vi "Chat_main.vi"() -> ()   [LabVIEW 2011]
uses:
  Controls/Stage.ctl
panel:
  in  "Port":u16=13078
  in  "Host IP":string="127.0.0.1"
  out "OnlineList":string[](array[string])
  in  "Create":bool
  in  "OffLine":bool
  in  "Link":bool
  out "linked":bool
  in  "Nickname":string
  in  "Send":bool
  in  "MsgBox":string
  out "C_Room":string
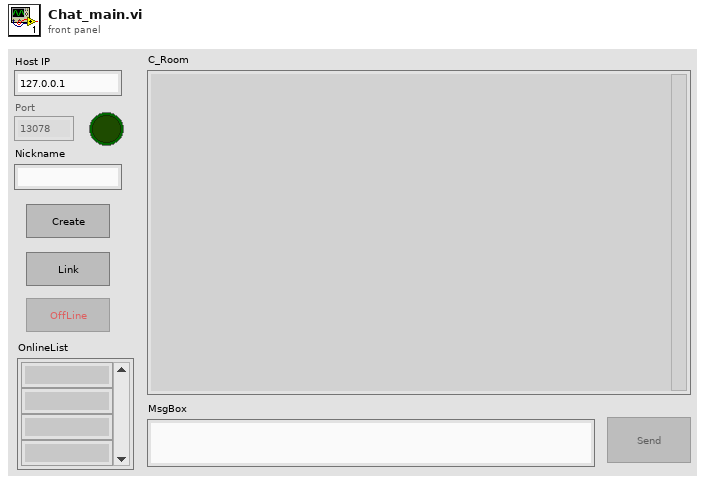
[diagram p1: front panel]
types:
  T1 = typedef "Stage.ctl" = enum16{"Initial", "Idle", "Link", "TX", "RX", "stop"}
  T2 = enum8{"Enabled", "Disabled", "Disabled and Grayed Out"}
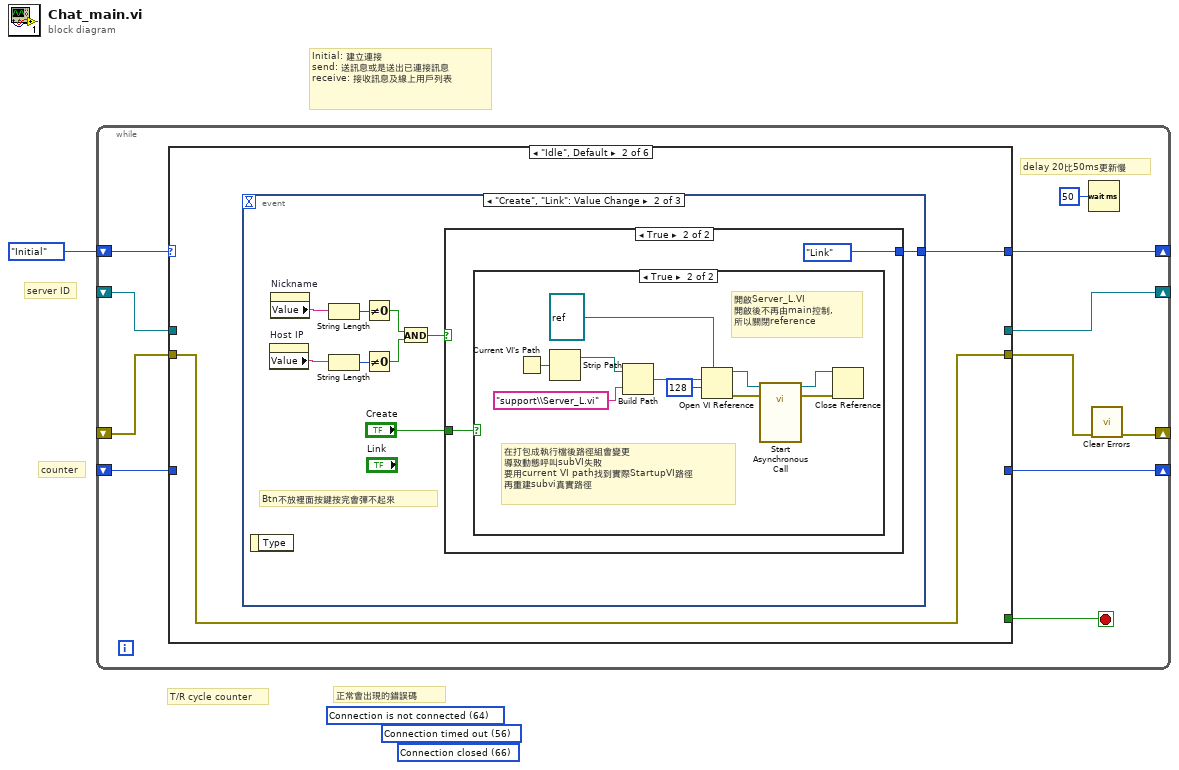
[diagram p0: block diagram]
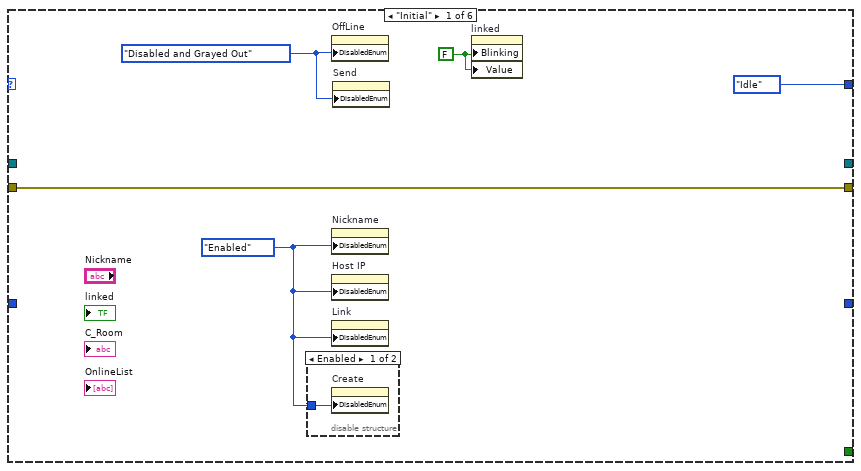
[diagram p2: hidden frame]
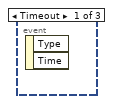
[diagram p4: hidden frame]
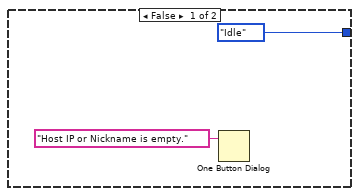
[diagram p5: hidden frame]
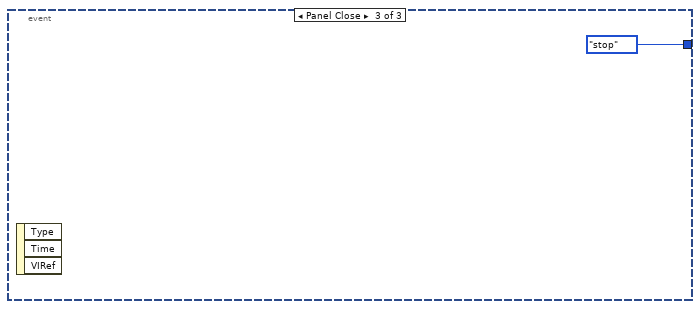
[diagram p7: hidden frame]
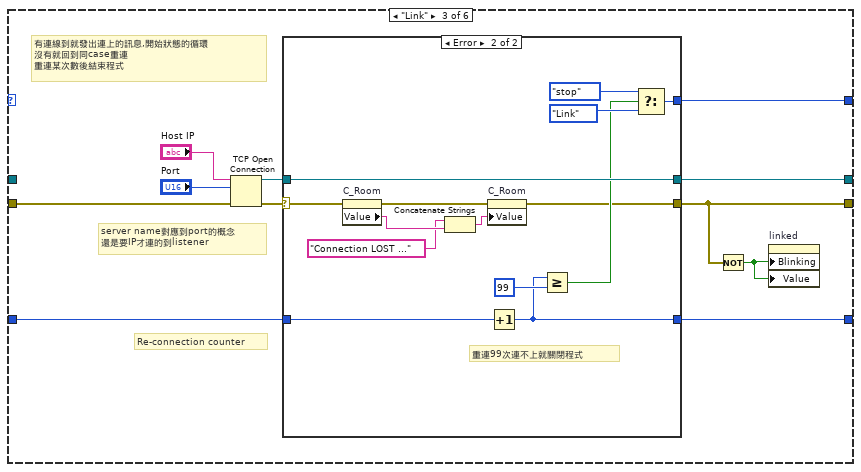
[diagram p8: hidden frame]
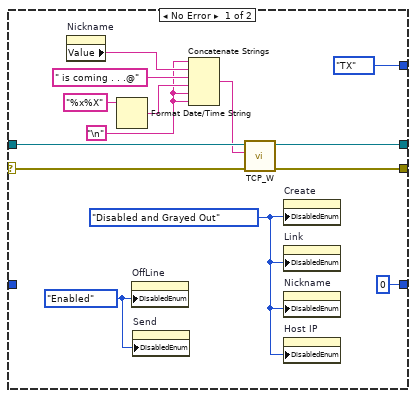
[diagram p9: hidden frame]
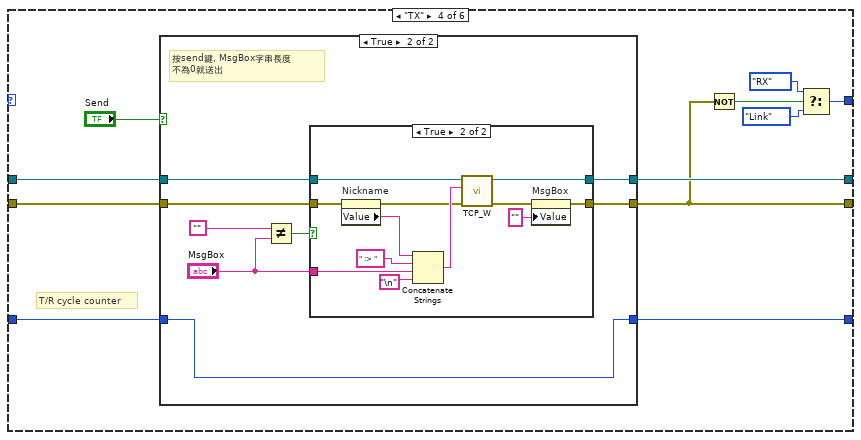
[diagram p10: hidden frame]
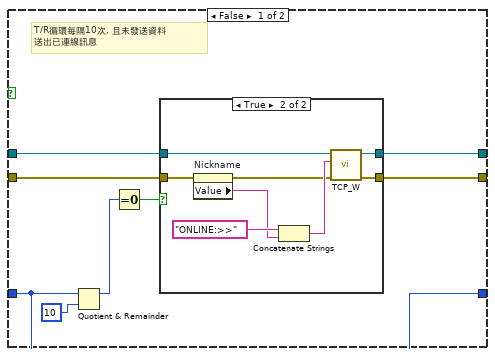
[diagram p11: hidden frame]
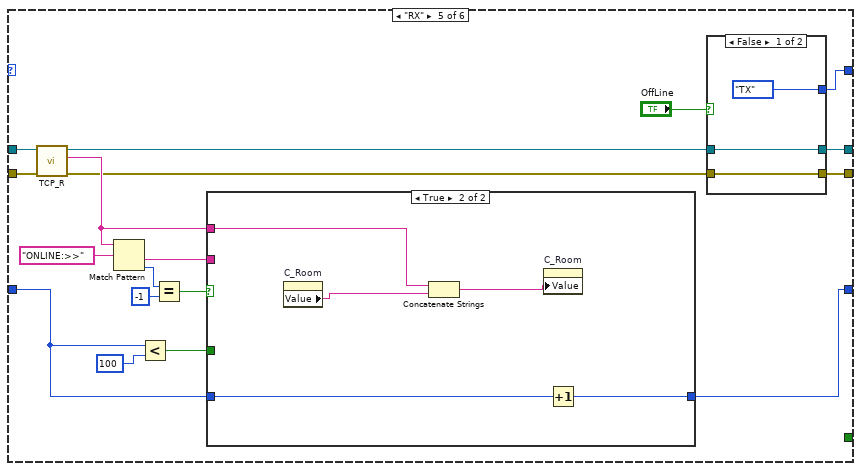
[diagram p14: hidden frame]
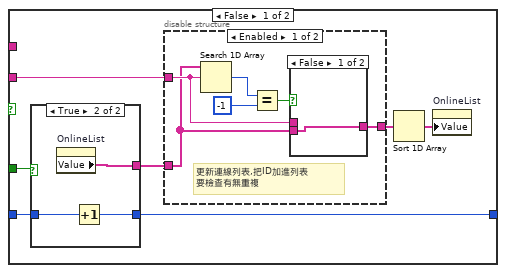
[diagram p15: hidden frame]
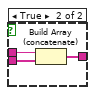
[diagram p16: hidden frame]
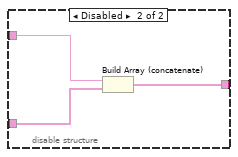
[diagram p17: hidden frame]
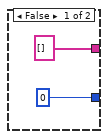
[diagram p18: hidden frame]
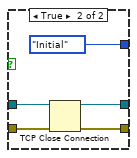
[diagram p19: hidden frame]
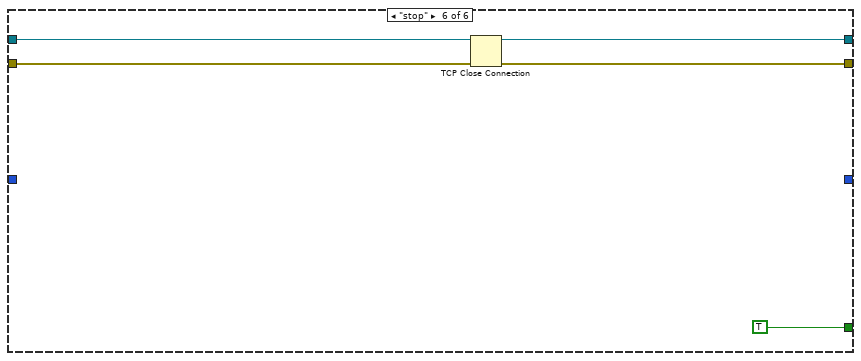
[diagram p20: hidden frame]
diagram:
  (unwired) 56 items=["No Error", "Argument Error", "Memory Full", "Out of Zone", "End of File", "File Already Open", "Generic File IO Error", "File Not Found", "File Permission Error", "Disk Full", "Duplicate Path", "Too Many Files Open", "Not Enabled", "Resource File Not Found", "Cannot Add Resource", "Resource Not Found", "Image Not Found", "Image Memory Error", "Pen Does Not Exist", "Config Bad Type", "Config Token Not Found", "Config Parse Error", "Config Memory Error", "Bad External Code Format", "Bad External Code Offset", "External Code Not Present", "Null Window", "Destroy Window Mixup", "Null Menu", "Print Aborted", "Bad Print Record", "Print Driver Error", "Windows Error During Print", "Memory Error During Print", "Print Dialog Error", "Generic Print Error", "Invalid Device Refnum", "Device Not Found", "Device Parameter Error", "Device Unit Error", "Can't Open Device", "Device Call Aborted", "Generic Error", "Cancelled By User", "Object ID Too Low", "Object ID Too High", "Object Not In Heap", "Unknown Heap", "Bad DefProc ID", "DefProc Not In Table", "Message Out Of Range", "Null Method", "Unknown Message", "Manager Call Not Supported", "Bad address", "Connection In progress", "Connection timed out", "Connection is already in progress", "Network attribute not supported", "Network error", "Address in use", "System out of memory", "Connection aborted", "Connection refused", "Connection is not connected", "Connection is already connected", "Connection closed", "Initialize error (interapplication manager)", "Bad occurrence", "Wait on unbound occurrence handler", "Occurrence queue overflow", "Bad path", "Semaphore not signaled", "Unrecognized type (interapplication manager)"] ("2nd Error to Convert")
  (unwired) 66 items=["No Error", "Argument Error", "Memory Full", "Out of Zone", "End of File", "File Already Open", "Generic File IO Error", "File Not Found", "File Permission Error", "Disk Full", "Duplicate Path", "Too Many Files Open", "Not Enabled", "Resource File Not Found", "Cannot Add Resource", "Resource Not Found", "Image Not Found", "Image Memory Error", "Pen Does Not Exist", "Config Bad Type", "Config Token Not Found", "Config Parse Error", "Config Memory Error", "Bad External Code Format", "Bad External Code Offset", "External Code Not Present", "Null Window", "Destroy Window Mixup", "Null Menu", "Print Aborted", "Bad Print Record", "Print Driver Error", "Windows Error During Print", "Memory Error During Print", "Print Dialog Error", "Generic Print Error", "Invalid Device Refnum", "Device Not Found", "Device Parameter Error", "Device Unit Error", "Can't Open Device", "Device Call Aborted", "Generic Error", "Cancelled By User", "Object ID Too Low", "Object ID Too High", "Object Not In Heap", "Unknown Heap", "Bad DefProc ID", "DefProc Not In Table", "Message Out Of Range", "Null Method", "Unknown Message", "Manager Call Not Supported", "Bad address", "Connection In progress", "Connection timed out", "Connection is already in progress", "Network attribute not supported", "Network error", "Address in use", "System out of memory", "Connection aborted", "Connection refused", "Connection is not connected", "Connection is already connected", "Connection closed", "Initialize error (interapplication manager)", "Bad occurrence", "Wait on unbound occurrence handler", "Occurrence queue overflow", "Bad path", "Semaphore not signaled", "Unrecognized type (interapplication manager)"] ("3rd Error to Convert")
  (unwired) 64 items=["No Error", "Argument Error", "Memory Full", "Out of Zone", "End of File", "File Already Open", "Generic File IO Error", "File Not Found", "File Permission Error", "Disk Full", "Duplicate Path", "Too Many Files Open", "Not Enabled", "Resource File Not Found", "Cannot Add Resource", "Resource Not Found", "Image Not Found", "Image Memory Error", "Pen Does Not Exist", "Config Bad Type", "Config Token Not Found", "Config Parse Error", "Config Memory Error", "Bad External Code Format", "Bad External Code Offset", "External Code Not Present", "Null Window", "Destroy Window Mixup", "Null Menu", "Print Aborted", "Bad Print Record", "Print Driver Error", "Windows Error During Print", "Memory Error During Print", "Print Dialog Error", "Generic Print Error", "Invalid Device Refnum", "Device Not Found", "Device Parameter Error", "Device Unit Error", "Can't Open Device", "Device Call Aborted", "Generic Error", "Cancelled By User", "Object ID Too Low", "Object ID Too High", "Object Not In Heap", "Unknown Heap", "Bad DefProc ID", "DefProc Not In Table", "Message Out Of Range", "Null Method", "Unknown Message", "Manager Call Not Supported", "Bad address", "Connection In progress", "Connection timed out", "Connection is already in progress", "Network attribute not supported", "Network error", "Address in use", "System out of memory", "Connection aborted", "Connection refused", "Connection is not connected", "Connection is already connected", "Connection closed", "Initialize error (interapplication manager)", "Bad occurrence", "Wait on unbound occurrence handler", "Occurrence queue overflow", "Bad path", "Semaphore not signaled", "Unrecognized type (interapplication manager)"] ("1st Error to Convert")
  # "正常會出現的錯誤碼"
  # "T/R cycle counter"
  # "server ID"
  # "counter"
  # "Initial: 建立連接\nsend: 送訊息或是送出已連接訊息\nreceive: 接收訊息及線上用戶列表"
  n1 = while {
    shift-right: [w11] -> _
    shift-left: Stage."Initial" -> [w12]
    shift-right: [w9] -> _
    shift-left: _ -> [w8]
    shift-right: [w2] -> _
    shift-left: _ -> [w7]
    shift-right: [w4] -> _
    shift-left: _ -> [w5]
    stop <- w10 stop-if-true
    # "delay 20比50ms更新慢"
    n2 = case shown="\"Idle\", Default" w12 {
      tunnel: [Stage."Idle" w20 w52 w89 w147 _] -> w11
      tunnel: [_ _ _ _ _ TRUE ("stop")] -> w10
      tunnel: [_ _ w54 w93 w148 w191] -> w9
      tunnel: w8 -> [_ _ _ w94 w152 w194]
      tunnel: [w14 w19 w47 w84 w146 w193] -> w3
      tunnel: w7 -> [w14 w19 w48 w92 w151 w192]
      tunnel: w5 -> [_ _ w51 w86 w138 _]
      tunnel: [_ _ w50 w85 w140 _] -> w4
      frame "Initial" {
        w13 = T2."Enabled" ("Disabled")
        w15 = FALSE ("Link")
        w16 = T2."Disabled and Grayed Out" ("Disabled")
        n3 = disable-structure shown="Enabled" {
          disable-tunnel: w13 -> [w18 _]
          frame Enabled {
            n4 = property on="Create" class="Bool"("DisabledEnum"=w18) -> ()  [unwired: 2 in, 2 out]
          }
          frame Disabled {
          }
        }
        n5 = property on="OffLine" class="Bool"("DisabledEnum"=w16) -> ()  [unwired: 2 in, 2 out]
        n6 = property on="Nickname" class="Str"("DisabledEnum"=w13) -> ()  [unwired: 2 in, 2 out]
        n7 = property on="Host IP" class="Str"("DisabledEnum"=w13) -> ()  [unwired: 2 in, 2 out]
        n8 = property on="Link" class="Bool"("DisabledEnum"=w13) -> ()  [unwired: 2 in, 2 out]
        n9 = property on="Send" class="Bool"("DisabledEnum"=w16) -> ()  [unwired: 2 in, 2 out]
        n10 = property on="linked" class="Bool (strict)"("Blinking"=w15, "Value"=w15) -> ()  [unwired: 2 in, 2 out]
      }
      frame "Idle", Default {
        n11 = event shown="[1] \"Create\", \"Link\": Value Change" {
          selector: _ -> [_ _ _]
          dyn-events: _ -> [_ _ _]
          timeout: _ -> [_ _ _]
          tunnel: [_ w29 Stage."stop"] -> w20
          event Timeout {
            n12 = event-data() -> ()  [unwired: 1 in, 2 out]
          }
          event "Create", "Link": Value Change {
            # "Btn不放裡面按鍵按完會彈不起來"
            n13 = event-data() -> ()  [unwired: 1 in, 1 out]
            n14 = property on="Host IP" class="Str"() -> ("Value"=w22:string)  [unwired: 2 in, 2 out]
            n15 = property on="Nickname" class="Str"() -> ("Value"=w25:string)  [unwired: 2 in, 2 out]
            n16 = String Length(string=w25) -> (length=w28:i32)
            n17 = String Length(string=w22) -> (length=w26:i32)
            n18 = Not Equal To 0?(x=w28) -> (x != 0?=w24:bool)
            n19 = Not Equal To 0?(x=w26) -> (x != 0?=w23:bool)
            n20 = And(x=w24, y=w23) -> (x .and. y?=w27:bool)
            n21 = case shown="True" w27 {
              tunnel: [Stage."Idle" Stage."Link"] -> w29
              tunnel: "Create" -> [_ w32]
              frame False {
                n22 = One Button Dialog(message="Host IP or Nickname is empty.") -> ()  [unwired: 1 in, 1 out]
              }
              frame True {
                n23 = case shown="True" w32 {
                  frame False {
                  }
                  frame True {
                    # "在打包成執行檔後路徑組會變更\n導致動態呼叫subVI失敗\n要用current VI path找到實際StartupVI路徑\n再重建subvi真實路徑"
                    # "開啟Server_L.VI\n開啟後不再由main控制,\n所以關閉reference"
                    n24 = Current VI's Path() -> (path=w35:path)
                    n25 = Strip Path(path=w35) -> (stripped path=w34:path)  [unwired: 1 out]
                    n26 = Build Path(base path=w34, name or relative path="support\\Server_L.vi" ("vi path")) -> (appended path=w39:path)
                    n27 = Open VI Reference(type specifier VI Refnum (for type only)=refnum<vi> refnum, vi path=w39, options=128) -> (vi reference=w43:refnum<vi>, error out=w41:errorcluster)  [unwired: 3 in]
                    n28 = call-by-ref "Start Asynchronous Call"(reference=w43, error in=w41) -> (reference out=w36:refnum<vi>, error out=w37:errorcluster)  [unwired: 12 in]
                    n29 = Close Reference(reference=w36, error in (no error)=w37) -> ()  [unwired: 1 out]
                  }
                }
              }
            }
          }
          event Panel Close {
            n30 = event-data() -> ()  [unwired: 1 in, 3 out]
          }
        }
      }
      frame "Link" {
        # "Re-connection counter"
        # "server name對應到port的概念\n還是要IP才連的到listener"
        # "有連線到就發出連上的訊息,開始狀態的循環\n沒有就回到同case重連\n重連某次數後結束程式"
        n31 = TCP Open Connection(address="Host IP", remote port or service name="Port", error in (no error)=w48) -> (connection ID=w55:refnum<k5>, error out=w53:errorcluster)  [unwired: 2 in]
        n32 = case shown="Error" w53 {
          selector: w53 -> [w68 w73]
          tunnel: [w58 w71] -> w47
          tunnel: w55 -> [w69 w83]
          tunnel: [w59 w83] -> w54
          tunnel: [Stage."TX" w81] -> w52
          tunnel: w51 -> [_ w82]
          tunnel: [0 w77] -> w50
          frame No Error {
            w57 = T2."Disabled and Grayed Out" ("Disabled")
            w60 = T2."Enabled" ("Disabled")
            w56 = "\n"
            n33 = property on="Nickname" class="Str"() -> ("Value"=w61:string)  [unwired: 2 in, 2 out]
            n34 = Format Date/Time String(time format string (%c)="%x%X") -> (date/time string=w62:string)  [unwired: 2 in]
            n35 = property on="OffLine" class="Bool"("DisabledEnum"=w60) -> ()  [unwired: 2 in, 2 out]
            n36 = property on="Send" class="Bool"("DisabledEnum"=w60) -> ()  [unwired: 2 in, 2 out]
            n37 = Concatenate Strings(w56, w61, " is coming . . .@" ("data in"), w62, w56, w56) -> (w64:string)
            n38 = call "TCP_W.vi"("error in"=w68, "data in"=w64, "connection ID"=w69) -> ("error IO"=w58:errorcluster, "connection ID out"=w59:refnum<k5>)  [unwired: 7 in]
            n39 = property on="Create" class="Bool"("DisabledEnum"=w57) -> ()  [unwired: 2 in, 2 out]
            n40 = property on="Link" class="Bool"("DisabledEnum"=w57) -> ()  [unwired: 2 in, 2 out]
            n41 = property on="Nickname" class="Str"("DisabledEnum"=w57) -> ()  [unwired: 2 in, 2 out]
            n42 = property on="Host IP" class="Str"("DisabledEnum"=w57) -> ()  [unwired: 2 in, 2 out]
          }
          frame Error {
            # "重連99次連不上就關閉程式"
            n43 = property on="C_Room" class="Str"(error in=w73) -> (error out=w72:errorcluster, "Value"=w74:string)  [unwired: 1 in, 1 out]
            n44 = Concatenate Strings("Connection LOST ..." ("string"), w74) -> (w75:string)
            n45 = property on="C_Room" class="Str"(error in=w72, "Value"=w75) -> (error out=w71:errorcluster)  [unwired: 1 in, 1 out]
            n46 = Increment(x=w82) -> (x+1=w77:i32)
            n47 = Greater Or Equal?(x=w77, y=99) -> (x >= y?=w76:bool)
            n48 = Select(t=Stage."stop", s=w76, f=Stage."Link") -> (s? t:f=w81:T1)
          }
        }
        n49 = Not(x=w47) -> (.not. x?=w49:bool)
        n50 = property on="linked" class="Bool (strict)"("Blinking"=w49, "Value"=w49) -> ()  [unwired: 2 in, 2 out]
      }
      frame "TX" {
        # "T/R cycle counter"
        n51 = case shown="True" "Send" {
          tunnel: w94 -> [w102 w119]
          tunnel: [w101 w118] -> w93
          tunnel: w92 -> [w100 w120]
          tunnel: [w99 w117] -> w84
          tunnel: w86 -> [w95 w116]
          tunnel: [w95 w116] -> w85
          frame False {
            # "T/R循環每隔10次, 且未發送資料\n送出已連線訊息"
            n52 = Quotient & Remainder(x=w95, y=10) -> (x-y*floor(x/y)=w98:i32)  [unwired: 1 out]
            n53 = Equal To 0?(x=w98) -> (x = 0?=w96:bool)
            n54 = case shown="True" w96 {
              tunnel: w102 -> [w103 w112]
              tunnel: [w103 w111] -> w101
              tunnel: w100 -> [w104 w106]
              tunnel: [w104 w110] -> w99
              frame False {
              }
              frame True {
                n55 = property on="Nickname" class="Str"(error in=w106) -> (error out=w105:errorcluster, "Value"=w107:string)  [unwired: 1 in, 1 out]
                n56 = Concatenate Strings("ONLINE:>>" ("data in"), w107) -> (w108:string)
                n57 = call "TCP_W.vi"("error in"=w105, "data in"=w108, "connection ID"=w112) -> ("error IO"=w110:errorcluster, "connection ID out"=w111:refnum<k5>)  [unwired: 7 in]
              }
            }
          }
          frame True {
            # "按send鍵, MsgBox字串長度\n不為0就送出"
            n58 = Not Equal?(x="", y="MsgBox") -> (x != y?=w113:bool)
            n59 = case shown="True" w113 {
              tunnel: w119 -> [w121 w131]
              tunnel: w120 -> [w122 w124]
              tunnel: [w122 w128] -> w117
              tunnel: "MsgBox" -> [_ w126]
              tunnel: [w121 w125] -> w118
              frame False {
              }
              frame True {
                n60 = property on="Nickname" class="Str"(error in=w124) -> (error out=w123:errorcluster, "Value"=w127:string)  [unwired: 1 in, 1 out]
                n61 = Concatenate Strings(w127, " :> ", w126, "\n") -> (w132:string)
                n62 = call "TCP_W.vi"("error in"=w123, "data in"=w132, "connection ID"=w131) -> ("error IO"=w129:errorcluster, "connection ID out"=w125:refnum<k5>)  [unwired: 7 in]
                n63 = property on="MsgBox" class="Str"(error in=w129, "Value"="" ("MsgBox")) -> (error out=w128:errorcluster)  [unwired: 1 in, 1 out]
              }
            }
          }
        }
        n64 = Not(x=w84) -> (.not. x?=w88:bool)
        n65 = Select(t=Stage."RX", s=w88, f=Stage."Link") -> (s? t:f=w89:T1)
      }
      frame "RX" {
        n66 = call "TCP_R.vi"("error in"=w151, "connection ID"=w152) -> ("error out"=w135:errorcluster, "data out"=w136:string, "connection ID out"=w149:refnum<k5>)  [unwired: 7 in]
        n67 = Match Pattern(string=w136, regular expression="ONLINE:>>") -> (after substring=w141:string, offset past match=w142:i32)  [unwired: 1 in, 2 out]
        n68 = Less?(x=w138, y=100) -> (x < y?=w137:bool)
        n69 = Equal?(x=w142, y=-1 ("offset (0)")) -> (x = y?=w143:bool)
        n70 = case shown="True" w143 {
          tunnel: w136 -> [_ w180]
          tunnel: w141 -> [w159 _]
          tunnel: w138 -> [w155 w181]
          tunnel: [w158 w182] -> w140
          tunnel: w137 -> [w154 _]
          frame False {
            n71 = case shown="True" w154 {
              tunnel: [0 ("t") w177] -> w158
              tunnel: [string[] [] ("OnlineList") w175] -> w157
              tunnel: w155 -> [_ w176]
              frame False {
              }
              frame True {
                n72 = property on="OnlineList" class="Arr (strict)"() -> ("Value"=w175:string[])  [unwired: 2 in, 2 out]
                n73 = Increment(x=w176) -> (x+1=w177:i32)
              }
            }
            n74 = disable-structure shown="Enabled" {
              disable-tunnel: w159 -> [w162 w172]
              disable-tunnel: w157 -> [w161 w171]
              disable-tunnel: [w160 w170] -> w156
              frame Enabled {
                # "更新連線列表,把ID加進列表\n要檢查有無重複"
                n75 = Search 1D Array(1D array=w161, element=w162) -> (index of element=w163:i32)  [unwired: 1 in]
                n76 = Equal?(x=w163, y=-1) -> (x = y?=w164:bool)
                n77 = case shown="False" w164 {
                  tunnel: [w166 w169] -> w160
                  tunnel: w162 -> [_ w168]
                  tunnel: w161 -> [w166 w167]
                  frame False {
                  }
                  frame True {
                    n78 = Build Array (concatenate)(w168, w167) -> (w169:string[])
                  }
                }
              }
              frame Disabled {
                n79 = Build Array (concatenate)(w172, w171) -> (w170:string[])
              }
            }
            n80 = Sort 1D Array(array=w156) -> (sorted array=w153:string[])
            n81 = property on="OnlineList" class="Arr (strict)"("Value"=w153) -> ()  [unwired: 2 in, 2 out]
          }
          frame True {
            n82 = property on="C_Room" class="Str"() -> ("Value"=w178:string)  [unwired: 2 in, 2 out]
            n83 = Concatenate Strings(w180, w178) -> (w179:string)
            n84 = property on="C_Room" class="Str"("Value"=w179) -> ()  [unwired: 2 in, 2 out]
            n85 = Increment(x=w181) -> (x+1=w182:i32)
          }
        }
        n86 = case shown="False" "OffLine" {
          tunnel: [Stage."TX" Stage."Initial"] -> w147
          tunnel: w149 -> [w184 w189]
          tunnel: [w184 w188] -> w148
          tunnel: [w183 w187] -> w146
          tunnel: w135 -> [w183 w186]
          frame False {
          }
          frame True {
            n87 = TCP Close Connection(connection ID=w189, error in (no error)=w186) -> (connection ID out=w188:refnum<k5>, error out=w187:errorcluster)  [unwired: 1 in]
          }
        }
      }
      frame "stop" {
        n88 = TCP Close Connection(connection ID=w194, error in (no error)=w192) -> (connection ID out=w191:refnum<k5>, error out=w193:errorcluster)  [unwired: 1 in]
      }
    }
    n89 = Wait (ms)(milliseconds to wait=u32 50) -> ()  [unwired: 1 out]
    n90 = call <vilib>:"Clear Errors.vi"("error in (no error)"=w3) -> ("error out"=w2:errorcluster)  [unwired: 5 in, 1 out]
  }
